vi "Contour Line_Main (1D).vi"(6 "number of heights":i32, 8 "Heights":dbl[](array[numeric]), 9 "Z":dbl[][](array[numeric]), 10 "Y":dbl[][](array[numeric]), 11 "X":dbl[][](array[numeric])) -> (2 "Contour Line":T1[](array[typedef]), 3 "Contour Graph":cluster{dbl[], dbl[]}[](graph))   [LabVIEW 2020, in "NI_AAL_Geometry.lvlib"]
uses:
  <vilib>/Analysis/NI_AAL_Geometry.lvlib
  <vilib>/Analysis/geometry.llb/Contour Lines Control.ctl
  <vilib>/Analysis/geometry.llb/Contour Line Segment.ctl
panel:
  # "Contour Line"
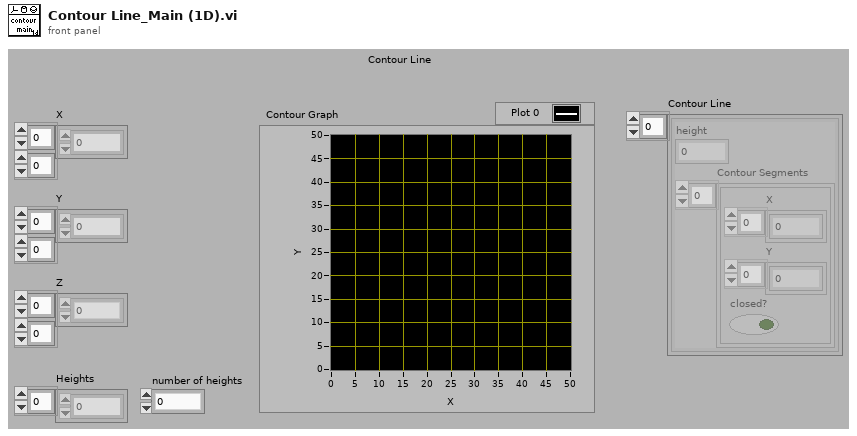
[diagram p1: front panel]
types:
  T1 = typedef "NI_AAL_Geometry.lvlib/Contour Lines Control.ctl" = cluster{"height":dbl, "Contour Segments":T2[]}
  T2 = typedef "NI_AAL_Geometry.lvlib/Contour Line Segment.ctl" = cluster{"X":dbl[], "Y":dbl[], "closed?":bool}
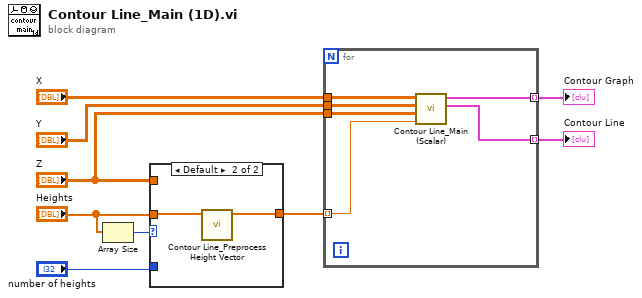
[diagram p0: block diagram]
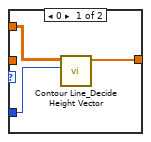
[diagram p2: hidden frame]
diagram:
  n1 = Array Size(array="Heights") -> (size(s)=w9:i32)
  n2 = case shown="Default" w9 {
    tunnel: "Z" -> [w12 _]
    tunnel: "number of heights" -> [w11 _]
    tunnel: "Heights" -> [_ w14]
    tunnel: [w10 w13] -> w8
    frame 0 {
      n3 = call <vilib>:"Contour Line_Decide Height Vector.vi"("number of heights"=w11, "Z"=w12) -> ("Height Vector"=w10:dbl[])  [unwired: 9 out]
    }
    frame Default {
      n4 = call <vilib>:"Contour Line_Preprocess Height Vector.vi"("Height Vector In"=w14) -> ("Height Vector Out"=w13:dbl[])  [unwired: 10 out]
    }
  }
  n5 = for {
    tunnel: w8 -> [w20] mode=indexing
    tunnel: "X" -> [w19]
    tunnel: "Y" -> [w17]
    tunnel: "Z" -> [w18]
    tunnel: [w16] -> w2 mode=indexing
    tunnel: [w15] -> w1 mode=indexing
    n6 = call <vilib>:"Contour Line_Main (Scalar).vi"("height"=w20, "Z"=w18, "Y"=w17, "X"=w19) -> ("Contour Line"=w16:T1, "Contour Graph"=w15:cluster{dbl[], dbl[]})  [unwired: 6 in]
  }
  "Contour Graph" <- w1
  "Contour Line" <- w2
